vi "Error.vi"(8 "error in":errorcluster, 10 "data":variant) -> (0 "error out":errorcluster)   [LabVIEW 2018, in "Controller.lvlib"]
doc: "This VI enqueues the named action"
uses:
  Controller.lvlib
  Private Controls/Module Data Cluster.ctl
  Private Controls/Module Action.ctl
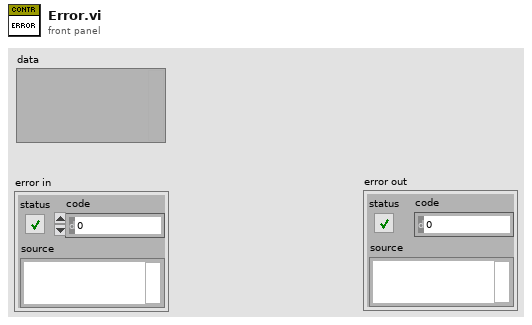
[diagram p1: front panel]
types:
  T1 = typedef "Controller.lvlib/Module Data Cluster.ctl" = cluster{"Variant":variant, "action":T2}
  T2 = typedef "Controller.lvlib/Module Action.ctl" = enum16{"error", "exit", "init", "start", "Under Body Wash", "Bug Remover", "Pre-Soak", "High Pressure", "Low PRessure Wax", "Spot Free Rinse", "Tire Shine Foam", "Air Dry", "Car Wash Complete", "Load Vehicle Position Array", "Vehicle Position", "Receive Config Data"}
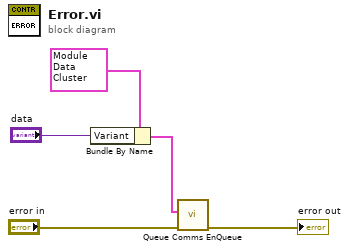
[diagram p0: block diagram]
diagram:
  n1 = Bundle By Name(cluster=T1 {"Variant"=variant, "action"=enum."error"} ("Module Data Cluster"), "Variant"="data") -> (w3:T1)
  n2 = call "Queue Comms EnQueue.vi"("error in"="error in", "Module Data Cluster"=w3) -> ("error out"=→"error out":errorcluster)  [unwired: 9 in]
